vi "Put Message.vi"(8 "error in (no error)":errorcluster, 9 "Message":string, 10 "Queue":string, 11 "Azure Session in":refnum<class "Session.lvclass">) -> (0 "error out":errorcluster, 2 "Message ID":string, 3 "Azure Session out":refnum<class "Session.lvclass">)   [LabVIEW 2015, in "NI_Azure_Queue.lvlib"]
doc: "Adds a message to the queue."
uses:
  NI_Azure_Queue.lvlib
  Core/Session/Session.lvclass
  Core/Signature Fields.ctl
  Core/Session/Session.lvclass/Session.ctl
  Core/Session/Write Request body.vi
  Core/Session/Write Request Parameters.vi
  Core/Session/Write HTTP Verb.vi
  Core/Session/Write URL Suffix.vi
  Core/Session/Write Signature Fields.vi
  Core/Name Value Pair.ctl
  Core/NI_Azure_Core.lvlib
  XML Parsing/NI_Azure_XML Parsing.lvlib
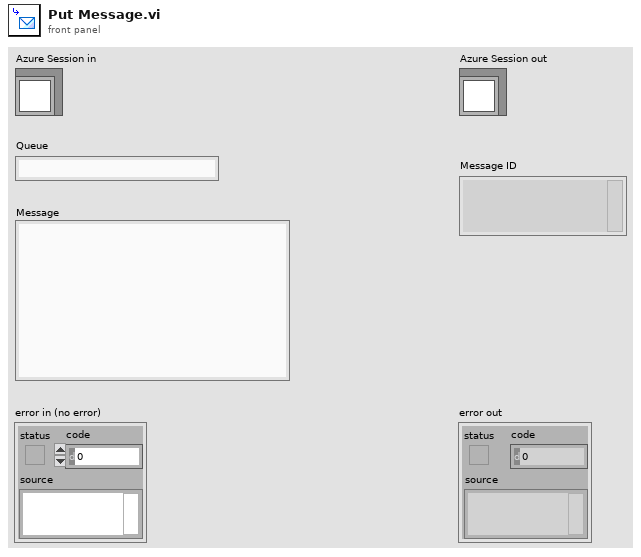
[diagram p1: front panel]
types:
  T1 = typedef "NI_Azure_Core.lvlib/Signature Fields.ctl" = cluster{"Content-Encoding":string, "Content-Language":string, "Content-Length":string, "Content-MD5":string, "Content-Type":string, "Date":string, "If-Modified-Since":string, "If-Match":string, "If-None-Match":string, "If-Unmodified-Since":string, "Range":string}
  T2 = typedef "NI_Azure_Core.lvlib/Name Value Pair.ctl" = cluster{"name":string, "value":string}
  T3 = typedef "NI_Azure_Core.lvlib/Response.ctl" = cluster{"Headers":string, "Body":string}
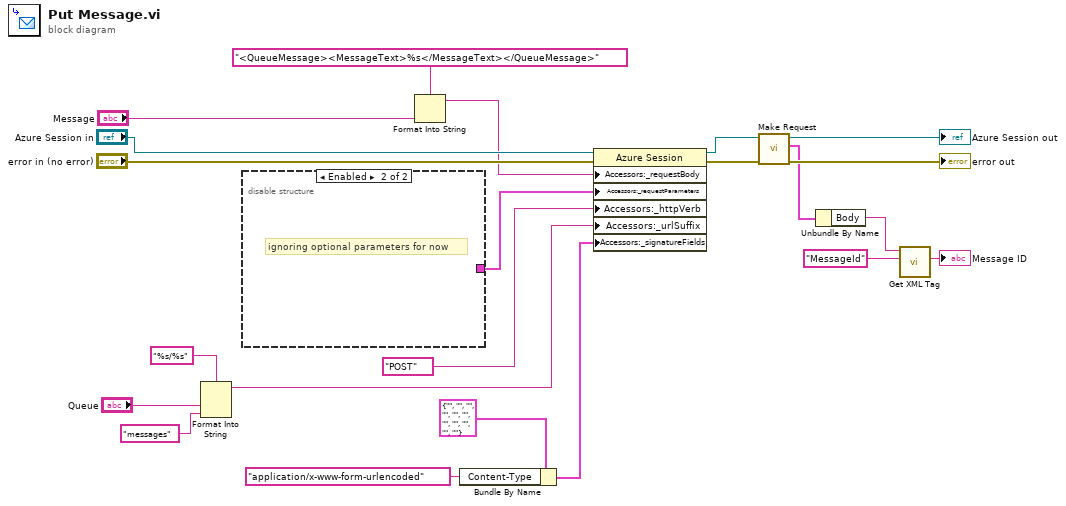
[diagram p0: block diagram]
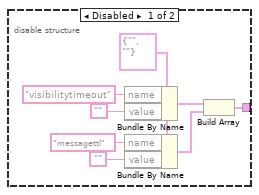
[diagram p2: hidden frame]
diagram:
  n1 = Format Into String(format string="%s/%s", "Queue", "messages") -> (resulting string=w8:string)  [unwired: 2 in, 1 out]
  n2 = disable-structure shown="Enabled" {
    disable-tunnel: [w30 _] -> w16
    frame Disabled {
      w28 = T2 {"name"="", "value"=""} ("Name Value Pair")
      n3 = Bundle By Name(cluster=w28, "name"="visibilitytimeout", "value"="") -> (w29:T2)
      n4 = Bundle By Name(cluster=w28, "name"="messagettl", "value"="") -> (w27:T2)
      n5 = Build Array(w29, w27) -> (w30:T2[])
    }
    frame Enabled {
      # "ignoring optional parameters for now"
    }
  }
  n6 = Format Into String(format string="<QueueMessage><MessageText>%s</MessageText></QueueMessage>", "Message") -> (resulting string=w13:string)  [unwired: 2 in, 1 out]
  n7 = Bundle By Name(cluster=T1 {"Content-Encoding"="", "Content-Language"="", "Content-Length"="", "Content-MD5"="", "Content-Type"="", "Date"="", "If-Modified-Since"="", "If-Match"="", "If-None-Match"="", "If-Unmodified-Since"="", "Range"=""} ("_signatureFields"), "Content-Type"="application/x-www-form-urlencoded") -> (w5:T1)
  n8 = property class="Azure Session"(reference="Azure Session in", error in="error in (no error)", "Accessors:_requestBody"=w13, "Accessors:_requestParameters"=w16, "Accessors:_httpVerb"="POST" ("HTTP-Verb"), "Accessors:_urlSuffix"=w8, "Accessors:_signatureFields"=w5) -> (reference out=w19:refnum<class "Session.lvclass">, error out=w17:errorcluster)
  n9 = call "Make Request.vi"("error in (no error)"=w17, "Session in"=w19) -> ("error out"=→"error out":errorcluster, "Response"=w4:T3, "Session out"=→"Azure Session out":refnum<class "Session.lvclass">)  [unwired: 7 in]
  n10 = Unbundle By Name(w4) -> ("Body"=w2:string)
  n11 = call "Get XML Tag.vi"("Tag name"="MessageId", "XML String in"=w2) -> ("Tag value"=→"Message ID":string)  [unwired: 5 in, 4 out]
